vi "Launch Topic.vi"(7 "Include Initial Value? (F)":bool, 9 "Type":variant, 10 "Datum Name":string, 11 "MonitoredMediator in":refnum<class "MonitoredMediator.lvclass">) -> (0 "error out":errorcluster, 2 "New Topic Enqueuer":refnum<class "Message Enqueuer.lvclass">, 3 "MonitoredMediator out":refnum<class "MonitoredMediator.lvclass">)   [LabVIEW 2020, in "MonitoredMediator.lvlib" / "MonitoredMediator.lvclass"]
uses:
  <vilib>/gpm_packages/@cs/mva-core/Source/MonitoredMediator/MonitoredMediator/MonitoredMediator.lvclass
  <vilib>/ActorFramework/Message Enqueuer/Message Enqueuer.lvclass
  <vilib>/gpm_packages/@cs/mva-core/Source/MonitoredMediator/MonitoredMediator/MonitoredMediator.lvclass/MonitoredMediator.ctl
  <vilib>/gpm_packages/@cs/mva-core/Source/MonitoredMediator/IBusMonitor/IBusMonitor.lvclass
  <vilib>/gpm_packages/@cs/mva-core/Source/Mediator/Topic Messages/Add Topic Subscriber Msg/Add Topic Subscriber Msg.lvclass/Add Topic Subscriber Msg.ctl
  <vilib>/ActorFramework/Message Enqueuer/Message Enqueuer.lvclass/Message Enqueuer.ctl
  <vilib>/ActorFramework/Message Enqueuer/Enqueue.vi
  <vilib>/gpm_packages/@cs/mva-core/Source/Mediator/Topic Messages/Add Topic Subscriber Msg/Add Topic Subscriber Msg.lvclass
  C:/Program Files/National Instruments/LabVIEW 2020/vi.lib/ActorFramework/Message/Message.lvclass
  <vilib>/ActorFramework/Message Priority Queue/Priority Enqueue.vi
  <vilib>/gpm_packages/@cs/mva-core/Source/Mediator/Mediator/Mediator.lvclass
  <vilib>/gpm_packages/@cs/mva-core/Source/IMediator/ISubscriptionPolicy/ISubscriptionPolicy.lvclass
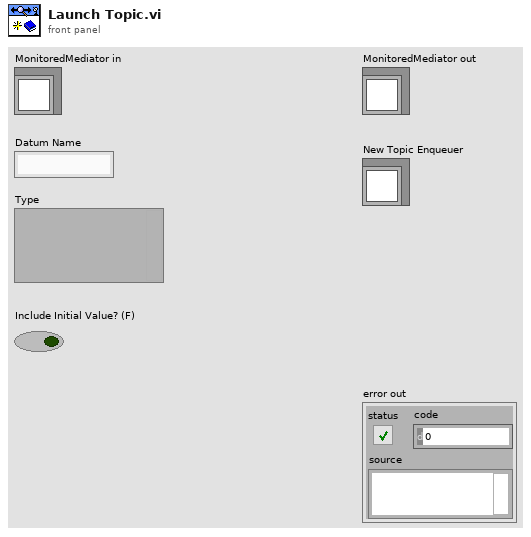
[diagram p1: front panel]
types:
  T1 = typedef "IMediator.lvlib/ISubscriptionPolicy.lvclass/ISubscriptionPolicy Reference.ctl" = refnum<data-value>
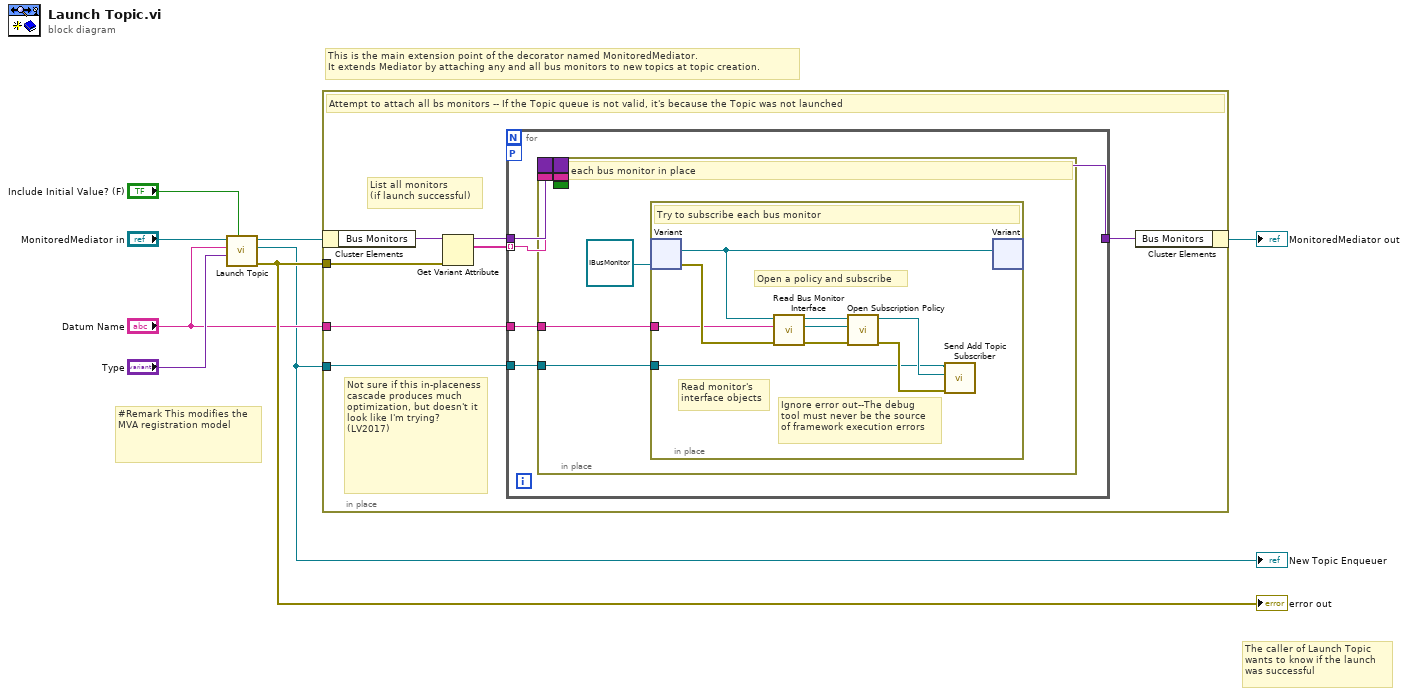
[diagram p0: block diagram]
diagram:
  # "#Remark This modifies the MVA registration model"
  # "The caller of Launch Topic\nwants to know if the launch\nwas successful"
  # "This is the main extension point of the decorator named MonitoredMediator.\nIt extends Mediator by attaching any and all bus monitors to new topics at topic creation."
  n1 = call-parent "Launch Topic.vi"("Include Initial Value? (F)"="Include Initial Value? (F)", "Type"="Type", "Datum Name"="Datum Name", "Mediator in"="MonitoredMediator in") -> ("error out"=w3:errorcluster, "New Topic Enqueuer"=w1:refnum<class "Message Enqueuer.lvclass">, "Mediator out"=w4:refnum<class "MonitoredMediator.lvclass">)  [unwired: 5 in]
  "error out" <- w3
  "New Topic Enqueuer" <- w1
  n2 = in-place {
    in-place-border: w1 -> [w9]
    in-place-border: w3 -> [w11]
    in-place-border: "Datum Name" -> [w10]
    # "Not sure if this in-placeness\ncascade produces much\noptimization, but doesn't it\nlook like I'm trying? (LV2017)"
    # "List all monitors\n(if launch successful)"
    # "Attempt to attach all bs monitors -- If the Topic queue is not valid, it's because the Topic was not launched"
    n3 = in-place-cluster #1(w4) -> ("Bus Monitors"=w14:variant)
    n4 = Get Variant Attribute(Variant=w14, error in=w11) -> (duplicate Variant=w13:variant, names=w12:string[])  [unwired: 2 in, 2 out]
    n5 = for {
      tunnel: [w20] -> w15
      tunnel: w13 -> [w19]
      tunnel: w12 -> [w18] mode=indexing
      tunnel: w10 -> [w17]
      tunnel: w9 -> [w16]
      workers-P: _ -> [_]
      n6 = in-place {
        border: w19 -> [_]
        border: w18 -> [_]
        border: [_] -> w20
        border: _ -> [_]
        border: _ -> [_]
        in-place-border: w17 -> [w22]
        in-place-border: w16 -> [w21]
        # "Read each bus monitor in place"
        n7 = in-place {
          in-place-border: w22 -> [w27]
          in-place-border: w21 -> [w26]
          # "Ignore error out--The debug\ntool must never be the source\nof framework execution errors"
          # "Open a policy and subscribe"
          # "Read monitor's\ninterface objects"
          # "Try to subscribe each bus monitor"
          n8 = in-place-variant #2(w25, refnum<class "IBusMonitor.lvclass"> refnum ("IBusMonitor")) -> (w29:refnum<class "IBusMonitor.lvclass">, w28:errorcluster)
          n9 = call-dynamic "Read Bus Monitor Interface.vi"("Datum Name"=w27, "IBusMonitor"=w29) -> ("Valid Transport"=w32:refnum<class "ITransport.lvclass">, "SubscriptionPolicy Type"=w33:refnum<class "ISubscriptionPolicy.lvclass">)  [unwired: 8 in]
          n10 = call <vilib>:"Open Subscription Policy.vi"("error in (no error)"=w28, "Transport"=w32, "SubscriptionPolicy"=w33) -> ("error out"=w30:errorcluster, "Subscription Policy"=w31:T1)  [unwired: 7 in]
          n11 = call <vilib>:"Send Add Topic Subscriber.vi"("error in (no error)"=w30, "Subscription Policy"=w31, "Message Enqueuer"=w26) -> ()  [unwired: 7 in, 2 out]
          n12 = in-place-variant #2(w29) -> (w24:variant)  [unwired: 1 out]
        }
      }
    }
    n13 = in-place-cluster #1("Bus Monitors"=w15) -> (→"MonitoredMediator out":refnum<class "MonitoredMediator.lvclass">)
  }
